vi "BRig_dataAnalog_iOccurrence.vi"() -> (2 "output_iOccurrence":i32)   [LabVIEW 2014]
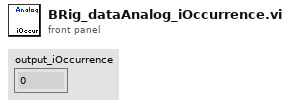
[diagram p1: front panel]
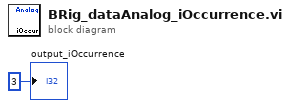
[diagram p0: block diagram]
diagram:
  "output_iOccurrence" <- 3 ("output_iBlock")
